vi "Configure Band Limiting Filter.vi"(5 "Enable Band Edge Low (T: Enable)":bool=TRUE, 6 "Band Edge Low (0 Hz)":dbl, 7 "Enable Band Edge High (T: Enable)":bool=TRUE, 8 "error in (no error)":errorcluster, 9 "Band Edge High (0 Hz)":dbl, 10 "Analyzer (0: A0)":i32(ring) items=["A0", "A1"], 11 "VISA resource name":refnum<visa-resource-name>) -> (0 "error out":errorcluster, 3 "VISA resource name out":refnum<visa-resource-name>)   [LabVIEW 2014, in "Stanford Research SR1.lvlib"]
doc: "Configures the attributes of the Band Limiting Filter."
uses:
  Stanford Research SR1.lvlib
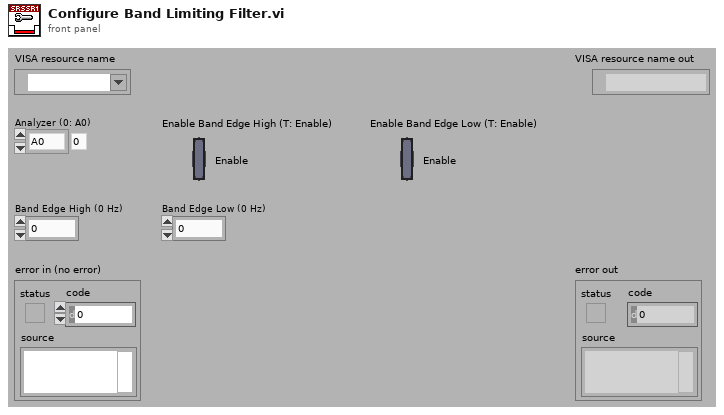
[diagram p1: front panel]
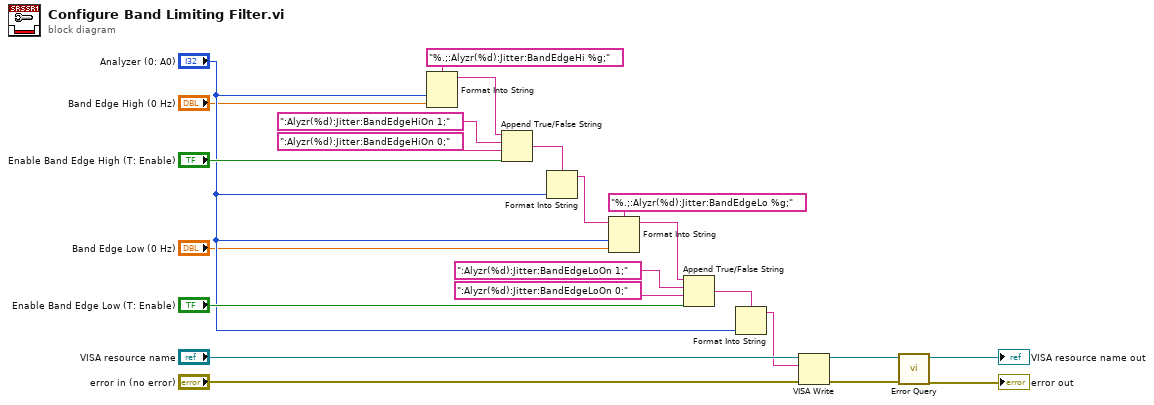
[diagram p0: block diagram]
diagram:
  n1 = Format Into String(format string="%.;:Alyzr(%d):Jitter:BandEdgeHi %g;", "Analyzer (0: A0)", "Band Edge High (0 Hz)") -> (resulting string=w22:string)  [unwired: 2 in, 1 out]
  n2 = Append True/False String(1:"Enable Band Edge High (T: Enable)", 2:":Alyzr(%d):Jitter:BandEdgeHiOn 0;", 3:":Alyzr(%d):Jitter:BandEdgeHiOn 1;", 4:w22) -> (0:w7:string)
  n3 = Format Into String(format string=w7, "Analyzer (0: A0)") -> (resulting string=w6:string)  [unwired: 2 in, 1 out]
  n4 = Format Into String(format string="%.;:Alyzr(%d):Jitter:BandEdgeLo %g;", initial string=w6, "Analyzer (0: A0)", "Band Edge Low (0 Hz)") -> (resulting string=w17:string)  [unwired: 1 in, 1 out]
  n5 = Append True/False String(1:"Enable Band Edge Low (T: Enable)", 2:":Alyzr(%d):Jitter:BandEdgeLoOn 0;", 3:":Alyzr(%d):Jitter:BandEdgeLoOn 1;", 4:w17) -> (0:w5:string)
  n6 = Format Into String(format string=w5, "Analyzer (0: A0)") -> (resulting string=w4:string)  [unwired: 2 in, 1 out]
  n7 = VISA Write(VISA resource name="VISA resource name", write buffer=w4, error in (no error)="error in (no error)") -> (VISA resource name out=w11:refnum<visa-resource-name>, error out=w10:errorcluster)  [unwired: 1 out]
  n8 = call "Error Query.vi"("error in (no error)"=w10, "VISA resource name"=w11) -> ("error out"=→"error out":errorcluster, "VISA resource name out"=→"VISA resource name out":refnum<visa-resource-name>)  [unwired: 6 in, 2 out]
